vi "MReadRS232_1.vi"(0 "port1":i32=9, 1 "dev1":i32=1, 4 "port2":i32=9, 5 "dev2":i32=2, 7 "port3":i32=13, 8 "dev7":i32=5, 9 "dev8":i32, 10 "port7":i32=12, 11 "port8":i32, 12 "dev5":i32=5, 14 "port5":i32=10, 15 "dev4":i32=4, 16 "dev6":i32=5, 17 "port6":i32=11, 18 "port4":i32=13, 19 "dev3":i32=3) -> (13 "params":dbl[](array[numeric]))   [LabVIEW 2015]
uses:
  BERTTA.dll
panel:
  # "MReadRS232(9, 1, 9, 2, 13, 3, 13, 4, 10, 5, 11, 5, 12, 5, 0, 0, res_vec);"
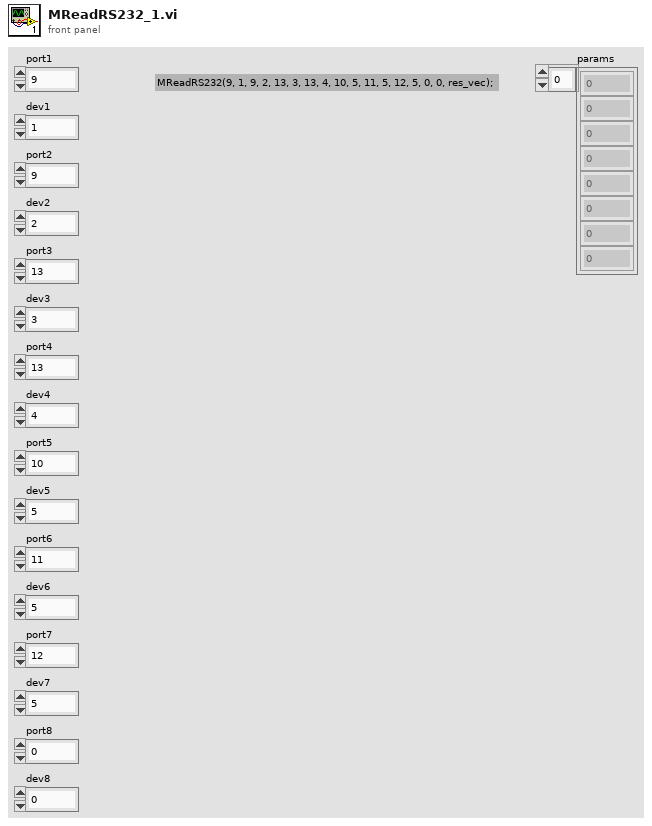
[diagram p1: front panel]
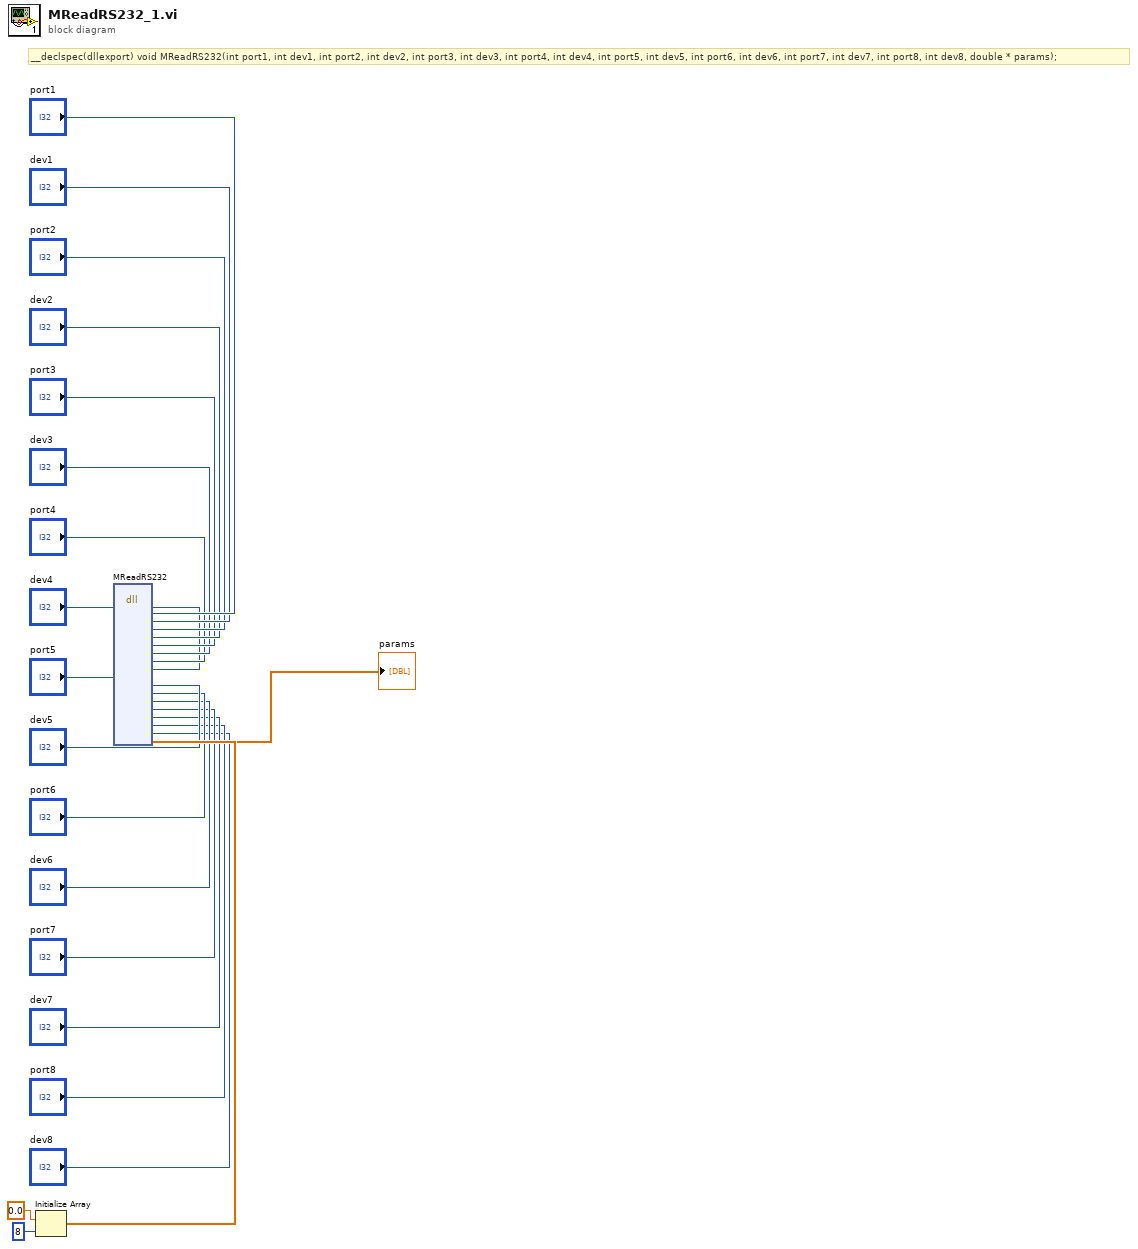
[diagram p0: block diagram]
diagram:
  # "__declspec(dllexport) void MReadRS232(int port1, int dev1, int port2, int dev2, int port3, int dev3, int port4, int dev4, int port5, int dev5, int port6, int dev6, int port7, int dev7, int port8, int dev8, double * params);"
  n1 = Initialize Array(0.0 ("element"), 8 ("dimension size")) -> (w20:dbl[])
  n2 = dll-call lib="C:/Users/shresplab/OneDrive - Kemira Oyj/Documents/Visual Studio 2017/Projects/Bertta/BERTTA/x64/Debug/BERTTA.dll" fn="MReadRS232"("port1"="port1", "dev1"="dev1", "port2"="port2", "dev2"="dev2", "port3"="port3", "dev3"="dev3", "port4"="port4", "dev4"="dev4", "port5"="port5", "dev5"="dev5", "port6"="port6", "dev6"="dev6", "port7"="port7", "dev7"="dev7", "port8"="port8", "dev8"="dev8", "params"=w20) -> ("params"=→"params":dbl[])  [unwired: 20 in, 2 out]
